vi "Configure Coupling.vi"(8 "error in (no error)":errorcluster, 10 "Coupling Setting (1: All)":u16(ring)=1 items=["None", "All", "Channels 1 & 2", "Channels 1 & 3", "Channels 2 & 3"], 11 "VISA resource name":refnum<visa-resource-name>) -> (0 "error out":errorcluster, 3 "VISA resource name out":refnum<visa-resource-name>)   [LabVIEW 2009, in "Agilent E363X Series.lvlib"]
doc: "Configures a defined coupling between various logical outputs of the power supply. Coupled outputs will be triggered simultaneously once a trigger is sent.\n\n<B>Note:</B> Only supported on E3631"
uses:
  <instrlib>/Agilent E363X Series/Agilent E363X Series.lvlib
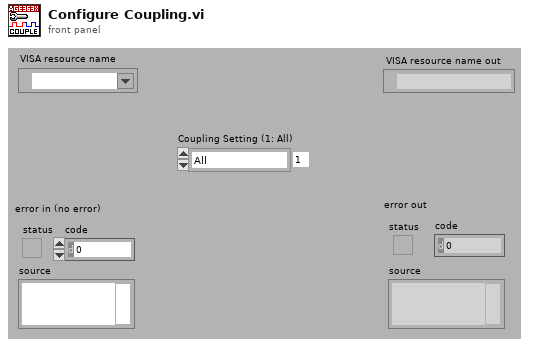
[diagram p1: front panel]
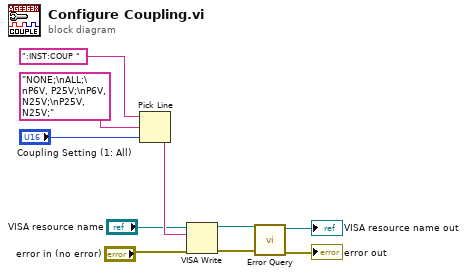
[diagram p0: block diagram]
diagram:
  n1 = Pick Line(string ("")=":INST:COUP ", multi-line string="NONE;\nALL;\nP6V, P25V;\nP6V, N25V;\nP25V, N25V;", line index="Coupling Setting (1: All)") -> (output string=w7:string)
  n2 = VISA Write(VISA resource name="VISA resource name", write buffer=w7, error in (no error)="error in (no error)") -> (VISA resource name out=w4:refnum<visa-resource-name>, error out=w3:errorcluster)  [unwired: 1 out]
  n3 = call <instrlib>:"Error Query.vi"("error in (no error)"=w3, "VISA resource name"=w4) -> ("error out"=→"error out":errorcluster, "VISA resource name out"=→"VISA resource name out":refnum<visa-resource-name>)  [unwired: 6 in, 2 out]
